vi "np_extraction_by_index_2d.vi"(10 "index array":i32[](array[numeric]), 11 "Array in":dbl[][](array[numeric])) -> (3 "Array out":dbl[][](array[numeric]))   [LabVIEW 2017]
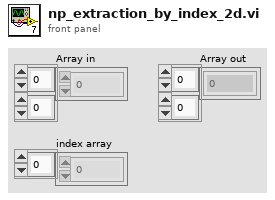
[diagram p1: front panel]
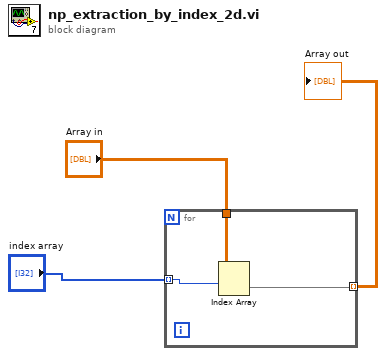
[diagram p0: block diagram]
diagram:
  n1 = for {
    tunnel: "index array" -> [w5] mode=indexing
    tunnel: "Array in" -> [w6]
    tunnel: [w4] -> w3 mode=indexing
    n2 = Index Array(array=w6, index (row)=w5) -> (element=w4:dbl[])  [unwired: 1 in]
  }
  "Array out" <- w3
